vi "load_parameters.vi"(4 "Create Data Folder (T)":bool=TRUE, 5 "Set Up Projector and Camera (T)":bool=TRUE, 6 "additional loaded parameters to write":string[][](array[string]), 8 "error in (no error)":errorcluster, 9 "StimulusObject Parameters":variant, 10 "StimulusObjectClassInput":refnum<class "StimulusObject.lvclass">, 11 "Tags":string) -> (0 "error out":errorcluster, 2 "Computer Found":bool, 3 "Parameters":T1 {"FW_WormLengthSD" format="%#.6f"})   [LabVIEW 2019]
uses:
  Parameters.ctl
  StimulusObject.lvclass
  <vilib>/AdvancedString/Delimited String to 1D String Array.vi
  ParametersGlobal.vi
  <vilib>/Utility/file.llb/Write Delimited Spreadsheet (string).vi
  <vilib>/vision/driver/NI_Vision_Acquisition_Software.lvlib
  <vilib>/vision/NI_Vision_Development_Module.lvlib
panel:
  out "Cores Utilized":u32
  out "Camera Frame Rate":dbl
  # "Faux Worm Drawing"
  # "Tracking"
  # "Temporal Calibration"
  # "Stimulus Generation"
  # "Median Filtering"
  # "Experimental Settings"
  # "Camera and Projector Settings"
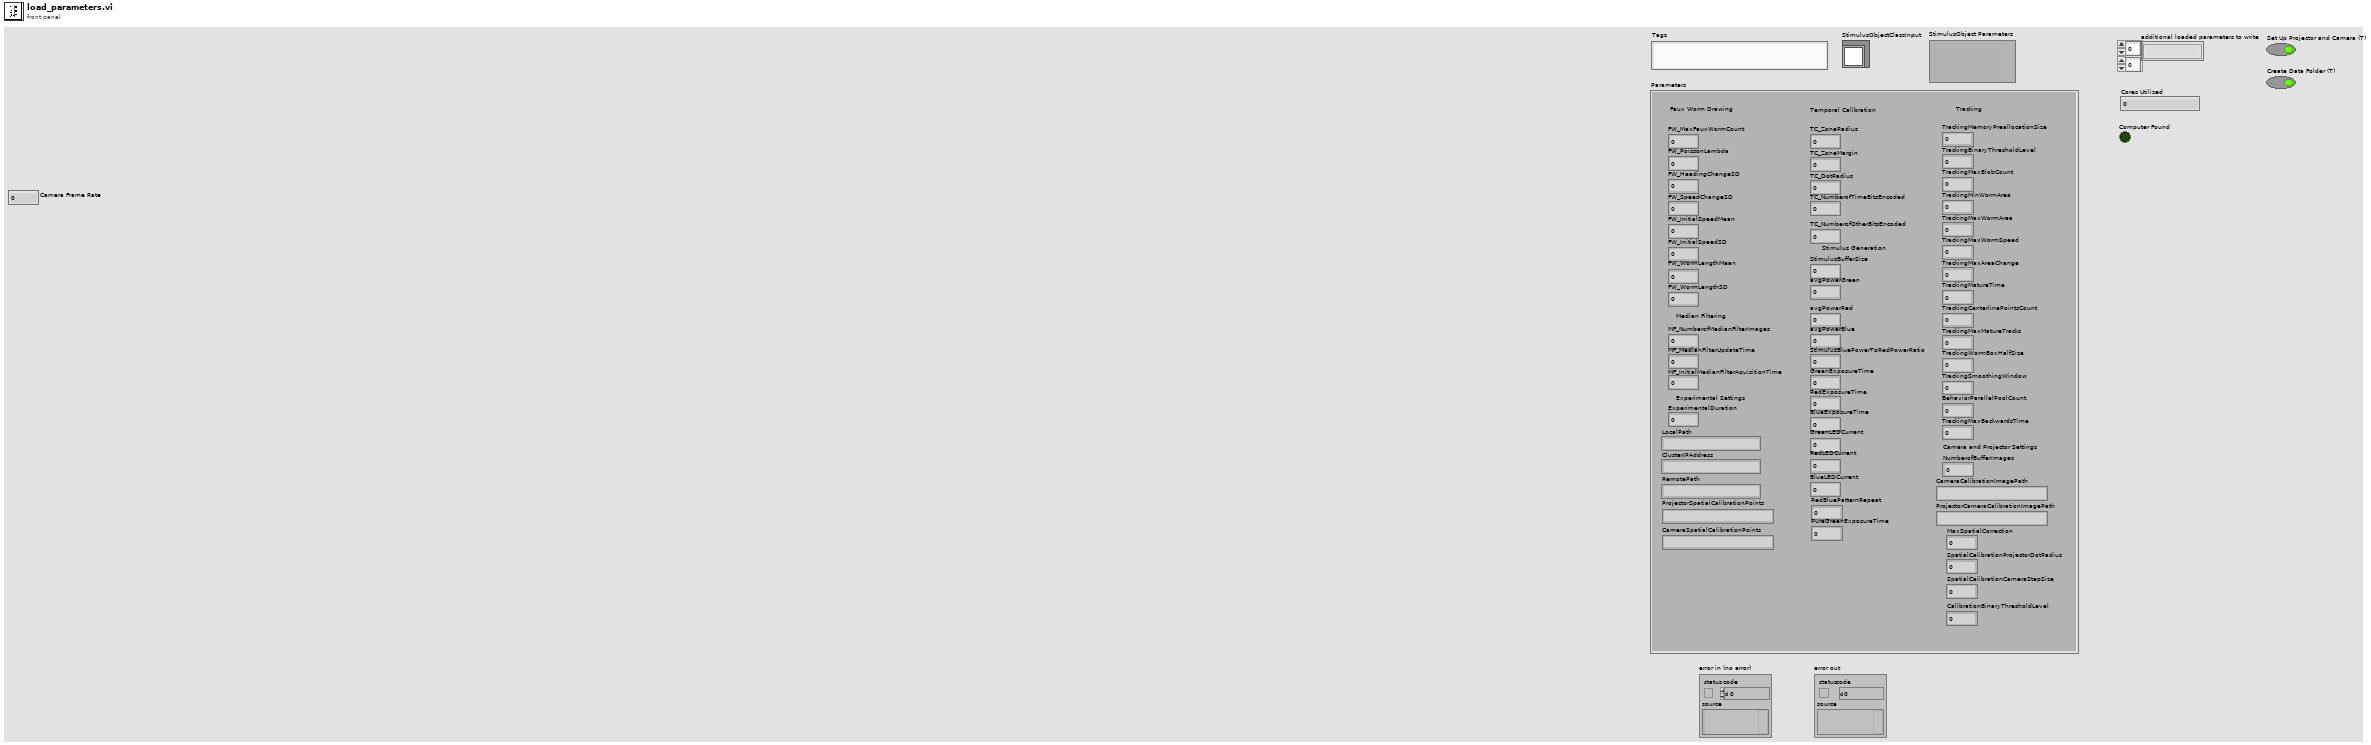
[diagram p1: front panel]
types:
  T1 = typedef "Parameters.ctl" = cluster{"FW_MaxFauxWormCount":i32, "FW_PoissonLambda":dbl, "FW_HeadingChangeSD":dbl, "FW_SpeedChangeSD":dbl, "FW_InitialSpeedMean":dbl, "FW_InitialSpeedSD":dbl, "FW_WormLengthMean":dbl, "FW_WormLengthSD":dbl, "MF_NumberofMedianFilterImages":i32, "MF_MedianFilterUpdateTime":i32, "MF_InitialMedianFilterAquisitionTime":dbl, "ExperimentalDuration":i32, "TC_ZoneRadius":i32, "TC_ZoneMargin":i32, "TC_DotRadius":dbl, "TC_NumberofTimeBitsEncoded":i32, "TC_NumberofOtherBitsEncoded":i32, "NumberofBufferImages":sgl, "CameraCalibrationImagePath":string, "ProjectorCameraCalibrationImagePath":string, "StimulusBufferSize":i32, "TrackingMemoryPreallocationSize":i32, "TrackingBinaryThresholdLevel":sgl, "TrackingMaxBlobCount":i32, "TrackingMinWormArea":dbl, "TrackingMaxWormArea":dbl, "TrackingMaxWormSpeed":dbl, "TrackingMaxAreaChange":dbl, "TrackingMatureTime":i32, "TrackingCenterlinePointsCount":i32, "TrackingMaxMatureTracks":i32, "TrackingWormBoxHalfSize":i32, "TrackingSmoothingWindow":i32, "BehaviorParallelPoolCount":i32, "LocalPath":string, "GreenExposureTime":i32, "RedExposureTime":i32, "BlueExposureTime":i32, "ClusterIPAddress":string, "RemotePath":string, "GreenLEDCurrent":u8, "RedLEDCurrent":u8, "BlueLEDCurrent":u8, "avgPowerGreen":sgl, "avgPowerRed":sgl, "avgPowerBlue":sgl, "StimulusBluePowerToRedPowerRatio":sgl, "TrackingMaxBackwardsTime":i32, "MaxSpatialCorrection":dbl, "ProjectorSpatialCalibrationPoints":string, "SpatialCalibrationProjectorDotRadius":i32, "SpatialCalibrationCameraStepSize":dbl, "CameraSpatialCalibrationPoints":string, "CalibrationBinaryThresholdLevel":dbl, "RedBluePatternRepeat":i32, "PureGreenExposureTime":i32}
  T2 = enum16{"open", "replace", "create", "open or create", "replace or create", "replace or create with confirmation"}
  T3 = typedef "IMAQ Image.ctl" = refnum<image>
  T4 = cluster{"Type":u32, "Version":u32, "Flags":u32, "SerialNumberHigh":u32, "SerialNumberLow":u32, "BusType":u32, "InterfaceName":string, "VendorName":string, "ModelName":string, "CameraFileName":string, "CameraAttributeURL":string}[]
  T5 = cluster{"Type":u32, "Version":u32, "Flags":u32, "SerialNumberHigh":u32, "SerialNumberLow":u32, "BusType":u32, "InterfaceName":string, "VendorName":string, "ModelName":string, "CameraFileName":string, "CameraAttributeURL":string}
  T6 = typedef "Image Type" = u32
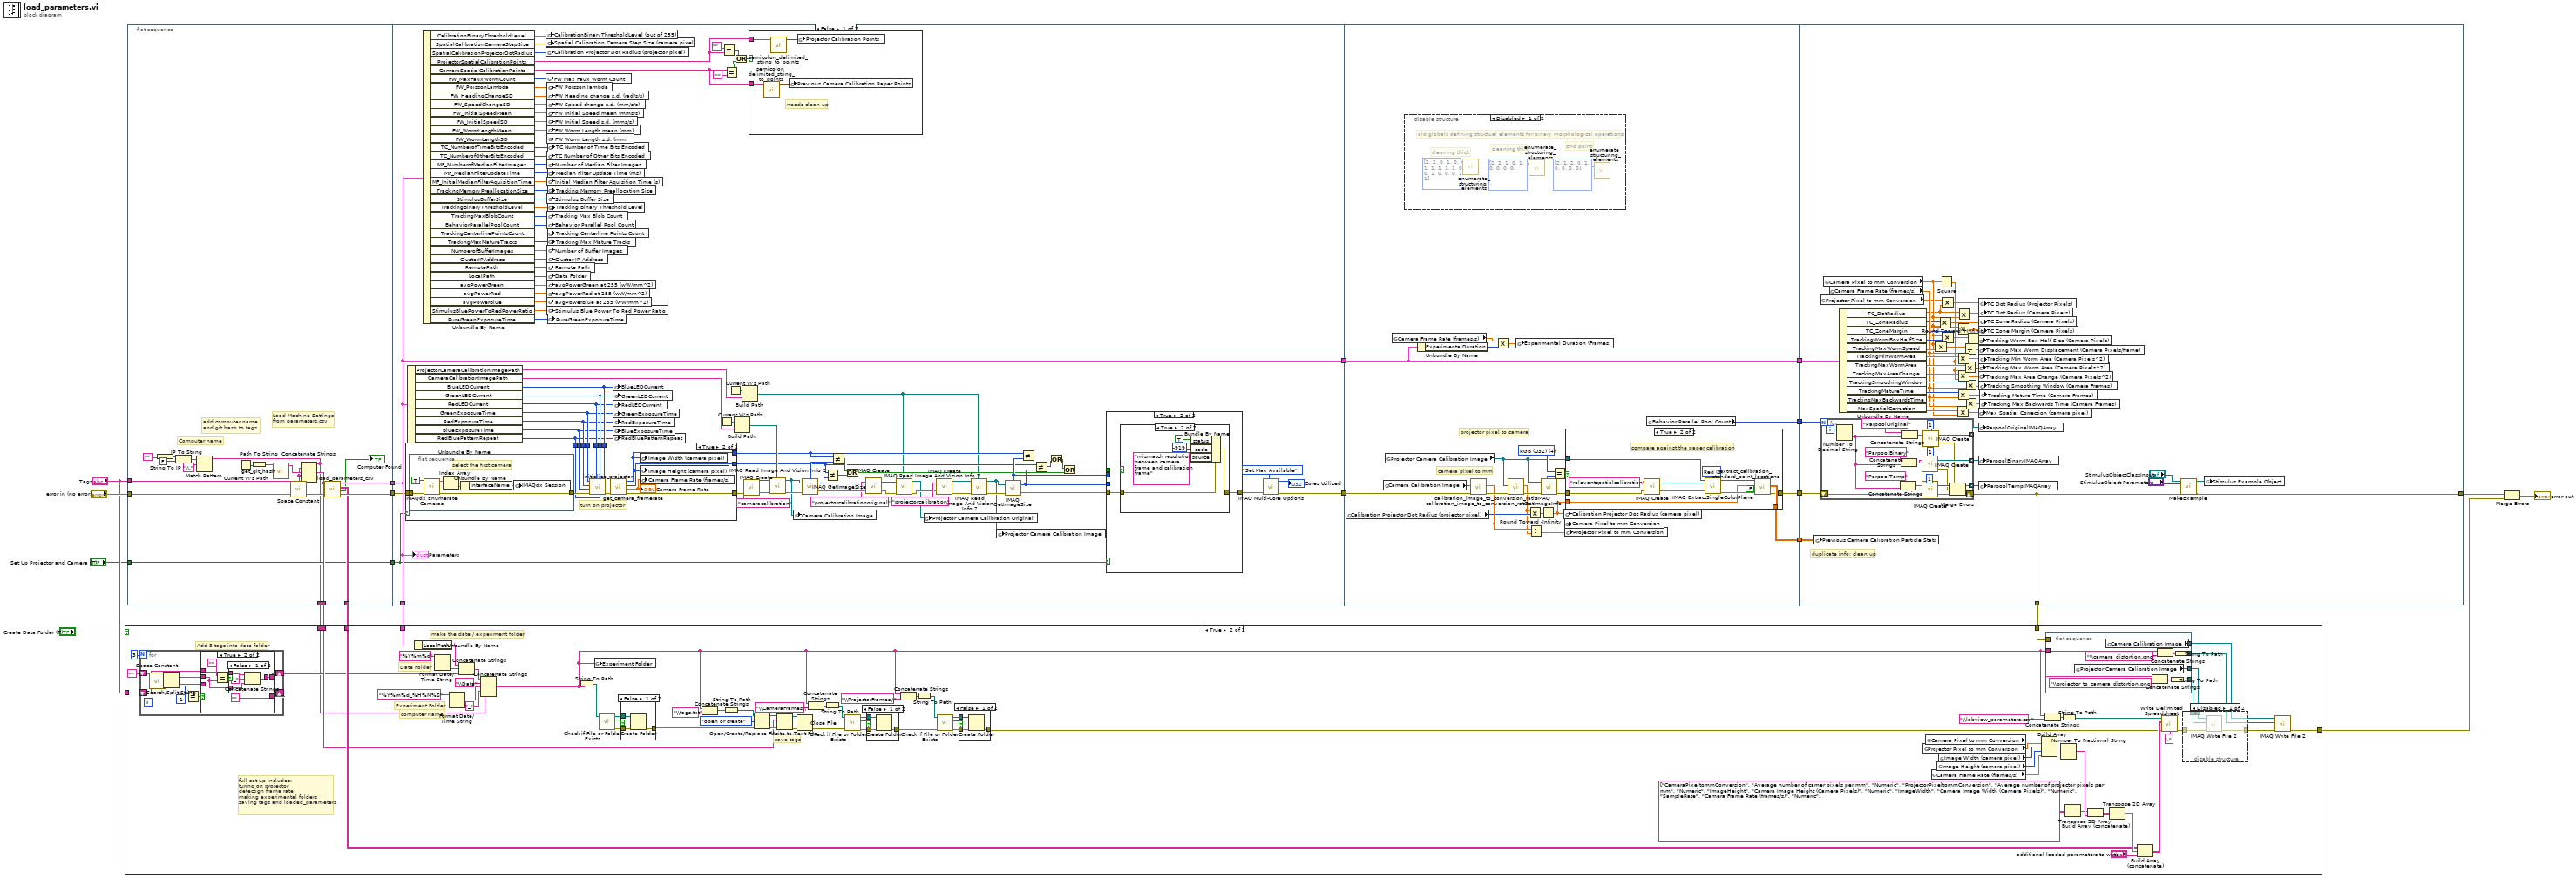
[diagram p0: block diagram]
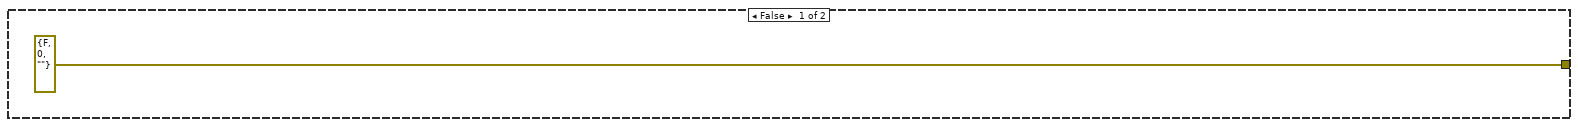
[diagram p2: hidden frame]
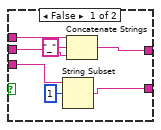
[diagram p7: hidden frame]
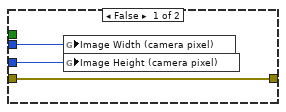
[diagram p10: hidden frame]
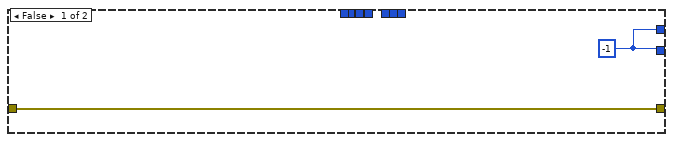
[diagram p12: hidden frame]
diagram:
  n1 = case shown="True" "Create Data Folder (T)" {
    tunnel: "Tags" -> [_ w92]
    tunnel: w12 -> [_ w41]
    tunnel: w11 -> [_ w39]
    tunnel: [errorcluster {"status"=FALSE, "code"=0, "source"=""} ("error out") w32] -> w8
    tunnel: w7 -> [_ w36]
    tunnel: w3 -> [_ w25]
    tunnel: w1 -> [_ w23]
    frame False {
    }
    frame True {
      # "computer name"
      # "full set up includes:\nturing on projector\ndetectign frame rate\nmaking experimental folders\nsaving tags and loaded_parameters"
      # "save tags"
      # "make the date / experiment folder"
      # "Experiment Folder"
      # "Date Folder"
      # "Add 3 tags into date folder"
      n2 = for {
        N: 3 -> [_]
        shift-right: [w119] -> _
        shift-left: w92 -> [w128]
        shift-right: [w121] -> w35
        shift-left: "" -> [w126]
        n3 = call <vilib>:"Space Constant.vi"() -> ("String"=w127:string)
        n4 = Search/Split String(string=w128, search string/char (-)=w127) -> (substring before match=w125:string, match + rest of string=w124:string, offset of match=w123:i32)  [unwired: 1 in]
        n5 = Equal?(x=w123, y=-1) -> (x = y?=w120:bool)
        n6 = case shown="True" w120 {
          tunnel: w126 -> [w129 w139]
          tunnel: w125 -> [w130 w136]
          tunnel: w124 -> [w131 _]
          tunnel: [w133 ""] -> w119
          tunnel: [w132 w138] -> w121
          frame False {
            n7 = String Subset(string=w131, offset (0)=1) -> (substring=w133:string)  [unwired: 1 in]
            n8 = Concatenate Strings(w129, "_", w130) -> (w132:string)
          }
          frame True {
            n9 = Equal?(x="", y=w136) -> (x = y?=w140:bool)
            n10 = case shown="False" w140 {
              tunnel: w139 -> [w143 w146]
              tunnel: [w144 w146] -> w138
              tunnel: w136 -> [w142 _]
              frame False {
                n11 = Concatenate Strings(w143, "_", w142) -> (w144:string)
              }
              frame True {
              }
            }
          }
        }
      }
      n12 = Unbundle By Name(w36) -> ("LocalPath"=w26:string)
      n13 = Format Date/Time String(time format string (%c)="%Y%m%d") -> (date/time string=w87:string)  [unwired: 2 in]
      n14 = Format Date/Time String(time format string (%c)="%Y%m%d_%H%M%S") -> (date/time string=w86:string)  [unwired: 2 in]
      n15 = Concatenate Strings(w26, w87, w35) -> (w88:string)
      n16 = Concatenate Strings(w88, "\\Data", w86, "_", w23) -> (w27:string)
      n17 = String To Path(string=w27) -> (path=w85:path)
      n18 = global write "ParametersGlobal.vi" "Experiment Folder"(w27) -> ()
      n19 = call <vilib>:"Check if File or Folder Exists.vi"("path"=w85) -> ("error out"=w89:errorcluster, "file or folder exists?"=w83:bool, "dup path"=w84:path)  [unwired: 8 in]
      n20 = case shown="False" w83 {
        tunnel: w84 -> [w117 _]
        tunnel: [w116 w118] -> w65
        tunnel: w89 -> [w115 w118]
        frame False {
          n21 = Create Folder(path (use dialog)=w117, error in=w115) -> (error out=w116:errorcluster)  [unwired: 1 in, 2 out]
        }
        frame True {
        }
      }
      n22 = Concatenate Strings(w27, "\\tags.txt" ("string")) -> (w69:string)
      n23 = String To Path(string=w69) -> (path=w72:path)
      n24 = Open/Create/Replace File(file path (use dialog)=w72, error in=w65, operation (0:open)=T2."open or create") -> (refnum out=w71:refnum<file>, error out=w70:errorcluster)  [unwired: 3 in, 1 out]
      n25 = Write to Text File(file (use dialog)=w71, text=w39, error in=w70) -> (refnum out=w73:refnum<file>, error out=w74:errorcluster)  [unwired: 1 in, 1 out]
      n26 = Close File(refnum=w73, error in=w74) -> (error out=w77:errorcluster)  [unwired: 1 out]
      n27 = Concatenate Strings(w27, "\\CameraFrames\\" ("string")) -> (w78:string)
      n28 = String To Path(string=w78) -> (path=w79:path)
      n29 = call <vilib>:"Check if File or Folder Exists.vi"("error in (no error)"=w77, "path"=w79) -> ("error out"=w80:errorcluster, "file or folder exists?"=w76:bool, "dup path"=w75:path)  [unwired: 7 in]
      n30 = case shown="False" w76 {
        tunnel: w75 -> [w113 _]
        tunnel: [w112 w114] -> w40
        tunnel: w80 -> [w111 w114]
        frame False {
          n31 = Create Folder(path (use dialog)=w113, error in=w111) -> (error out=w112:errorcluster)  [unwired: 1 in, 2 out]
        }
        frame True {
        }
      }
      n32 = Concatenate Strings(w27, "\\ProjectorFrames\\" ("string")) -> (w61:string)
      n33 = String To Path(string=w61) -> (path=w62:path)
      n34 = call <vilib>:"Check if File or Folder Exists.vi"("error in (no error)"=w40, "path"=w62) -> ("error out"=w63:errorcluster, "file or folder exists?"=w60:bool, "dup path"=w59:path)  [unwired: 7 in]
      n35 = case shown="False" w60 {
        tunnel: w59 -> [w109 _]
        tunnel: [w108 w110] -> w38
        tunnel: w63 -> [w107 w110]
        frame False {
          n36 = Create Folder(path (use dialog)=w109, error in=w107) -> (error out=w108:errorcluster)  [unwired: 1 in, 2 out]
        }
        frame True {
        }
      }
      n37 = global read "ParametersGlobal.vi" "Projector Pixel to mm Conversion"() -> (w49:sgl)
      n38 = global read "ParametersGlobal.vi" "Camera Pixel to mm Conversion"() -> (w48:sgl)
      n39 = global read "ParametersGlobal.vi" "Camera Frame Rate (frames/s)"() -> (w64:sgl)
      n40 = global read "ParametersGlobal.vi" "Image Height (camera pixel)"() -> (w51:i32)
      n41 = global read "ParametersGlobal.vi" "Image Width (camera pixel)"() -> (w50:i32)
      n42 = Build Array(w48, w49, w50, w51, w64) -> (w52:sgl[])
      n43 = Concatenate Strings(w27, "\\labview_parameters.csv" ("string")) -> (w46:string)
      n44 = flat-sequence {
        tunnel: [w106] -> w31
        tunnel: [w105] -> w30
        tunnel: [w100] -> w29
        tunnel: [w99] -> w28
        tunnel: w27 -> [w98]
        tunnel: w25 -> [_]
        frame #0 {
          n45 = global read "ParametersGlobal.vi" "Projector Camera Calibration Image"() -> (w106:T3)
          n46 = global read "ParametersGlobal.vi" "Camera Calibration Image"() -> (w105:T3)
          n47 = Concatenate Strings(w98, "\\projector_to_camera_distortion.png" ("string")) -> (w102:string)
          n48 = Concatenate Strings(w98, "\\camera_distortion.png" ("string")) -> (w104:string)
          n49 = String To Path(string=w102) -> (path=w100:path)
          n50 = String To Path(string=w104) -> (path=w99:path)
        }
      }
      n51 = Number To Fractional String(number=w52) -> (F-format string=w54:string[])  [unwired: 3 in]
      n52 = String To Path(string=w46) -> (path=w47:path)
      n53 = Transpose 2D Array(2D array=string[][] [["CameraPixeltommConversion", "Average number of camer pixels per mm", "Numeric"], ["ProjectorPixeltommConversion", "Average number of projector pixels per mm", "Numeric"], ["ImageHeight", "Camera Image Height (Camera Pixels)", "Numeric"], ["ImageWidth", "Camera Image Width (Camera Pixels)", "Numeric"], ["SampleRate", "Camera Frame Rate (frames/s)", "Numeric"]]) -> (transposed array=w53:string[][])
      n54 = Build Array (concatenate)(w53, w54) -> (w55:string[][])
      n55 = Transpose 2D Array(2D array=w55) -> (transposed array=w56:string[][])
      n56 = Build Array (concatenate)(w41, w56, "additional loaded parameters to write") -> (w58:string[][])
      n57 = call-poly <vilib>:"Write Delimited Spreadsheet.vi"("file path (dialog if empty)"=w47, "2D data"=w58, "error in (no error)"=w38, "delimiter (\\t)"="," ("delimiter (\\t)")) -> ("error out"=w34:errorcluster)  [unwired: 10 in, 1 out]
      n58 = disable-structure shown="Disabled" {
        disable-tunnel: w34 -> [w96 w97]
        disable-tunnel: [w95 w97] -> w33
        disable-tunnel: w31 -> [w94 _]
        disable-tunnel: w29 -> [w93 _]
        frame Disabled {
          n59 = call-poly "IMAQ Write File 2"("error in (no error)"=w96, "File Path"=w93, "Image"=w94) -> ("error out"=w95:errorcluster)  [unwired: 7 in, 1 out]
        }
        frame Enabled {
        }
      }
      n60 = call-poly "IMAQ Write File 2"("error in (no error)"=w33, "File Path"=w28, "Image"=w30) -> ("error out"=w32:errorcluster)  [unwired: 7 in, 1 out]
    }
  }
  n61 = flat-sequence {
    tunnel: [w164] -> w20
    tunnel: "error in (no error)" -> [w150]
    tunnel: [w151] -> w19
    tunnel: "Tags" -> [w156]
    tunnel: [w153] -> w12
    tunnel: [w152] -> w11
    tunnel: [w149] -> w6
    tunnel: "Set Up Projector and Camera (T)" -> [w149]
    tunnel: [w147] -> w1
    tunnel: w20 -> [w222]
    tunnel: [w213] -> w18
    tunnel: w19 -> [w223]
    tunnel: [w223] -> w15
    tunnel: [w223] -> w7
    tunnel: w6 -> [w199]
    tunnel: w18 -> [w313]
    tunnel: [w301] -> w17
    tunnel: [w309] -> w16
    tunnel: w15 -> [w309]
    tunnel: [w310] -> w14
    tunnel: [w298] -> w2
    tunnel: w17 -> [w352]
    tunnel: w16 -> [w373]
    tunnel: w14 -> [w351]
    tunnel: [w340] -> w10
    tunnel: [w344] -> w3
    tunnel: w2 -> [w343]
    frame #0 {
      # "add computer name \nand git hash to tags"
      # "Computer name"
      # "Load Machine Settings\nfrom parameters.csv"
      n62 = String To IP(1:"") -> (0:w163:u32)
      n63 = IP To String(1:FALSE, 2:w163) -> (0:w160:string)
      n64 = Match Pattern(string=w160, regular expression="\\.") -> (before substring=w147:string)  [unwired: 1 in, 3 out]
      n65 = Current VI's Path() -> (path=w158:path)
      n66 = Path To String(path=w158) -> (string=w157:string)
      n67 = call "get_git_hash.vi"("VI folder"=w157) -> ("github hash"=w155:string)  [unwired: 10 in]
      n68 = call <vilib>:"Space Constant.vi"() -> ("String"=w154:string)
      n69 = Concatenate Strings(w147, w154, w155, w154, w156) -> (w152:string)
      n70 = call "load_parameters_csv.vi"("error in (no error)"=w150, "Tags In"=w152) -> ("error out"=w164:errorcluster, "Computer Found"=→"Computer Found":bool, "Loaded Params"=w153:string[][], "Parameters Out"=w151:T1)  [unwired: 6 in]
    }
    frame #1 {
      n71 = Unbundle By Name(w223) -> ("ProjectorCameraCalibrationImagePath"=w193:string, "CameraCalibrationImagePath"=w245:string, "BlueLEDCurrent"=w172:u8, "GreenLEDCurrent"=w171:u8, "RedLEDCurrent"=w170:u8, "GreenExposureTime"=w169:i32, "RedExposureTime"=w168:i32, "BlueExposureTime"=w167:i32, "RedBluePatternRepeat"=w166:i32)
      n72 = case shown="True" w199 {
        tunnel: w222 -> [w272 w277]
        tunnel: [w272 w284] -> w221
        tunnel: w169 -> [_ w283]
        tunnel: w168 -> [_ w282]
        tunnel: w167 -> [_ w281]
        tunnel: w170 -> [_ w280]
        tunnel: w172 -> [_ w279]
        tunnel: w171 -> [_ w278]
        tunnel: [w271 w275] -> w192
        tunnel: [w271 w274] -> w191
        tunnel: w166 -> [_ w273]
        frame False {
          w271 = -1 ("Image Width (camera pixel)")
        }
        frame True {
          # "turn on projector"
          n73 = flat-sequence {
            tunnel: w277 -> [w289]
            tunnel: [w288] -> w276
            frame #0 {
              # "select the first camera"
              n74 = call <vilib>:"IMAQdx Enumerate Cameras.vi"("error in"=w289, "Connected Only? (Yes)"=TRUE) -> ("error out"=w288:errorcluster, "Camera Information Array"=w292:T4)  [unwired: 8 in]
              n75 = Index Array(array=w292) -> (element=w291:T5)  [unwired: 1 in]
              n76 = Unbundle By Name(w291) -> ("InterfaceName"=w287:string)
              n77 = global write "ParametersGlobal.vi" "IMAQdx Session"(w287) -> ()
            }
          }
          n78 = call "initialize_projector.vi"("BlueCurrent"=w279, "RedBluePatternRepeat"=w273, "GreenCurrent"=w278, "RedCurrent"=w280, "error in"=w276, "blue exp_time_us"=w281, "red exp_time_us"=w282, "green exp_time_us"=w283) -> ("error out"=w285:errorcluster)  [unwired: 3 in]
          n79 = call "get_camera_framerate.vi"("error in"=w285) -> ("error out"=w284:errorcluster, "Camera Frame Rate"=w286:dbl, "Y Resolution"=w274:i32, "X Resolution"=w275:i32)  [unwired: 7 in]
          "Camera Frame Rate" <- w286
          n80 = global write "ParametersGlobal.vi" "Image Width (camera pixel)"(w275) -> ()
          n81 = global write "ParametersGlobal.vi" "Image Height (camera pixel)"(w274) -> ()
          n82 = global write "ParametersGlobal.vi" "Camera Frame Rate (frames/s)"(w286) -> ()
        }
      }
      n83 = Unbundle By Name(w223) -> ("CalibrationBinaryThresholdLevel"=w173:dbl, "SpatialCalibrationCameraStepSize"=w187:dbl, "SpatialCalibrationProjectorDotRadius"=w188:i32, "ProjectorSpatialCalibrationPoints"=w189:string, "CameraSpatialCalibrationPoints"=w174:string, "FW_MaxFauxWormCount"=w235:i32, "FW_PoissonLambda"=w236:dbl, "FW_HeadingChangeSD"=w237:dbl, "FW_SpeedChangeSD"=w238:dbl, "FW_InitialSpeedMean"=w239:dbl, "FW_InitialSpeedSD"=w240:dbl, "FW_WormLengthMean"=w241:dbl, "FW_WormLengthSD"=w242:dbl, "TC_NumberofTimeBitsEncoded"=w243:i32, "TC_NumberofOtherBitsEncoded"=w244:i32, "MF_NumberofMedianFilterImages"=w234:i32, "MF_MedianFilterUpdateTime"=w233:i32, "MF_InitialMedianFilterAquisitionTime"=w232:dbl, "TrackingMemoryPreallocationSize"=w231:i32, "StimulusBufferSize"=w230:i32, "TrackingBinaryThresholdLevel"=w229:sgl, "TrackingMaxBlobCount"=w228:i32, "BehaviorParallelPoolCount"=w227:i32, "TrackingCenterlinePointsCount"=w226:i32, "TrackingMaxMatureTracks"=w225:i32, "NumberofBufferImages"=w224:sgl, "ClusterIPAddress"=w220:string, "RemotePath"=w219:string, "LocalPath"=w218:string, "avgPowerGreen"=w214:sgl, "avgPowerRed"=w215:sgl, "avgPowerBlue"=w216:sgl, "StimulusBluePowerToRedPowerRatio"=w217:sgl, "PureGreenExposureTime"=w165:i32)
      n84 = global write "ParametersGlobal.vi" "CalibrationBinaryThresholdLevel (out of 255)"(w173) -> ()
      n85 = global write "ParametersGlobal.vi" "Spatial Calibration Camera Step Size (camera pixel)"(w187) -> ()
      n86 = global write "ParametersGlobal.vi" "Calibration Projector Dot Radius (projector pixel)"(w188) -> ()
      n87 = global write "ParametersGlobal.vi" "FW Max Faux Worm Count"(w235) -> ()
      n88 = global write "ParametersGlobal.vi" "FW Poisson lambda"(w236) -> ()
      n89 = global write "ParametersGlobal.vi" "FW Heading change s.d. (rad/s/s)"(w237) -> ()
      n90 = global write "ParametersGlobal.vi" "FW Speed change s.d. (mm/s/s)"(w238) -> ()
      n91 = global write "ParametersGlobal.vi" "FW Initial Speed mean (mms/s)"(w239) -> ()
      n92 = global write "ParametersGlobal.vi" "FW Initial Speed s.d. (mms/s)"(w240) -> ()
      n93 = global write "ParametersGlobal.vi" "FW Worm Length mean (mm)"(w241) -> ()
      n94 = global write "ParametersGlobal.vi" "FW Worm Length s.d. (mm)"(w242) -> ()
      n95 = global write "ParametersGlobal.vi" "TC Number of Other Bits Encoded"(w244) -> ()
      n96 = global write "ParametersGlobal.vi" "Number of Median Filter Images"(w234) -> ()
      n97 = global write "ParametersGlobal.vi" "Initial Median Filter Aquisition Time (s)"(w232) -> ()
      n98 = global write "ParametersGlobal.vi" "Stimulus Buffer Size"(w230) -> ()
      n99 = global write "ParametersGlobal.vi" "Tracking Max Blob Count"(w228) -> ()
      n100 = global write "ParametersGlobal.vi" "Behavior Parallel Pool Count"(w227) -> ()
      n101 = global write "ParametersGlobal.vi" "Number of Buffer Images"(w224) -> ()
      n102 = global write "ParametersGlobal.vi" "Cluster IP Address"(w220) -> ()
      n103 = global write "ParametersGlobal.vi" "Remote Path"(w219) -> ()
      n104 = global write "ParametersGlobal.vi" "Data Folder"(w218) -> ()
      n105 = global write "ParametersGlobal.vi" "avgPowerGreen at 255 (wW/mm^2)"(w214) -> ()
      n106 = global write "ParametersGlobal.vi" "avgPowerRed at 255 (wW/mm^2)"(w215) -> ()
      n107 = global write "ParametersGlobal.vi" "avgPowerBlue at 255 (wW/mm^2)"(w216) -> ()
      n108 = global write "ParametersGlobal.vi" "Stimulus Blue Power To Red Power Ratio"(w217) -> ()
      n109 = global write "ParametersGlobal.vi" "TC Number of Time Bits Encoded"(w243) -> ()
      n110 = global write "ParametersGlobal.vi" "Median Filter Update Time (ms)"(w233) -> ()
      n111 = global write "ParametersGlobal.vi" "Tracking Memory Preallocation Size"(w231) -> ()
      n112 = global write "ParametersGlobal.vi" "Tracking Binary Threshold Level"(w229) -> ()
      n113 = global write "ParametersGlobal.vi" "Tracking Centerline Points Count"(w226) -> ()
      n114 = global write "ParametersGlobal.vi" "Tracking Max Mature Tracks"(w225) -> ()
      n115 = global write "ParametersGlobal.vi" "PureGreenExposureTime"(w165) -> ()
      n116 = global write "ParametersGlobal.vi" "BlueLEDCurrent"(w172) -> ()
      n117 = global write "ParametersGlobal.vi" "GreenLEDCurrent"(w171) -> ()
      n118 = global write "ParametersGlobal.vi" "RedLEDCurrent"(w170) -> ()
      n119 = global write "ParametersGlobal.vi" "GreenExposureTime"(w169) -> ()
      n120 = global write "ParametersGlobal.vi" "RedExposureTime"(w168) -> ()
      n121 = global write "ParametersGlobal.vi" "BlueExposureTime"(w167) -> ()
      n122 = global write "ParametersGlobal.vi" "RedBluePatternRepeat"(w166) -> ()
      n123 = Current VI's Path() -> (path=w250:path)
      n124 = Equal?(x="", y=w189) -> (x = y?=w177:bool)
      n125 = Equal?(x=w174, y="") -> (x = y?=w176:bool)
      n126 = Current VI's Path() -> (path=w254:path)
      n127 = Or(x=w177, y=w176) -> (x .or. y?=w175:bool)
      n128 = Build Path(base path=w250, name or relative path=w245) -> (appended path=w247:path)
      n129 = Build Path(base path=w254, name or relative path=w193) -> (appended path=w180:path)
      n130 = call "IMAQ Create"("Image Name"="cameracalibration", "error in (no error)"=w221) -> ("New Image"=w249:T3, "error out"=w248:errorcluster)  [unwired: 3 in]
      n131 = case shown="False" w175 {
        tunnel: w189 -> [w258 _]
        tunnel: w174 -> [w256 _]
        frame False {
          # "needs clean up"
          n132 = call "semicolon_delimited_string_to_points.vi"("delimited string"=w256) -> ("Array"=w255:cluster{"X":dbl, "Y":dbl}[])  [unwired: 10 in]
          n133 = call "semicolon_delimited_string_to_points.vi"("delimited string"=w258) -> ("Array"=w257:cluster{"X":dbl, "Y":dbl}[])  [unwired: 10 in]
          n134 = global write "ParametersGlobal.vi" "Previous Camera Calibration Paper Points"(w255) -> ()
          n135 = global write "ParametersGlobal.vi" "Projector Calibration Points"(w257) -> ()
        }
        frame True {
        }
      }
      n136 = call "IMAQ Read Image And Vision Info 2"("File Path"=w247, "error in (no error)"=w248, "Image"=w249) -> ("error out"=w210:errorcluster, "Image Out"=w207:T3)  [unwired: 6 in, 1 out]
      n137 = global write "ParametersGlobal.vi" "Camera Calibration Image"(w207) -> ()
      n138 = call "IMAQ GetImageSize"("Image"=w207, "error in (no error)"=w210) -> ("Y Resolution"=w208:i32, "X Resolution"=w209:i32, "error out"=w185:errorcluster)  [unwired: 2 in]
      n139 = Not Equal?(x=w191, y=w208) -> (x != y?=w204:bool)
      n140 = Not Equal?(x=w192, y=w209) -> (x != y?=w203:bool)
      n141 = Or(x=w203, y=w204) -> (x .or. y?=w186:bool)
      n142 = call "IMAQ Create"("Image Name"="projectorcalibrationoriginal", "error in (no error)"=w185) -> ("New Image"=w182:T3, "error out"=w183:errorcluster)  [unwired: 3 in]
      n143 = call "IMAQ Read Image And Vision Info 2"("File Path"=w180, "error in (no error)"=w183, "Image"=w182) -> ("error out"=w181:errorcluster, "Image Out"=w179:T3)  [unwired: 6 in, 1 out]
      n144 = global write "ParametersGlobal.vi" "Projector Camera Calibration Original"(w179) -> ()
      n145 = call "IMAQ Create"("Image Name"="projectorcalibration", "error in (no error)"=w181) -> ("New Image"=w252:T3, "error out"=w251:errorcluster)  [unwired: 3 in]
      n146 = call "IMAQ Read Image And Vision Info 2"("File Path"=w180, "error in (no error)"=w251, "Image"=w252) -> ("error out"=w206:errorcluster, "Image Out"=w205:T3)  [unwired: 6 in, 1 out]
      n147 = global write "ParametersGlobal.vi" "Projector Camera Calibration Image"(w205) -> ()
      n148 = call "IMAQ GetImageSize"("Image"=w205, "error in (no error)"=w206) -> ("Y Resolution"=w196:i32, "X Resolution"=w195:i32, "error out"=w198:errorcluster)  [unwired: 2 in]
      n149 = Not Equal?(x=w192, y=w195) -> (x != y?=w202:bool)
      n150 = Not Equal?(x=w191, y=w196) -> (x != y?=w201:bool)
      n151 = Or(x=w202, y=w201) -> (x .or. y?=w200:bool)
      n152 = Or(x=w200, y=w186) -> (x .or. y?=w194:bool)
      n153 = case shown="True" w199 {
        tunnel: w198 -> [w261 w263]
        tunnel: [w261 w262] -> w197
        tunnel: w196 -> [w260 _]
        tunnel: w195 -> [w259 _]
        tunnel: w194 -> [_ w264]
        frame False {
          n154 = global write "ParametersGlobal.vi" "Image Width (camera pixel)"(w259) -> ()
          n155 = global write "ParametersGlobal.vi" "Image Height (camera pixel)"(w260) -> ()
        }
        frame True {
          n156 = case shown="True" w264 {
            tunnel: w263 -> [w265 w267]
            tunnel: [w265 w266] -> w262
            frame False {
              # "all resolutions match"
            }
            frame True {
              n157 = Bundle By Name(cluster=w267, "status"=TRUE, "code"=-919, "source"="mismatch resolution between camera frame and calibration frame") -> (w266:errorcluster)
            }
          }
        }
      }
      n158 = call "IMAQ Multi-Core Options"("Get/Set Number of Cores (Get)"=enum32{"Get", "Set", "Set Max Available"}."Set Max Available", "error in (no error)"=w197) -> ("error out"=w213:errorcluster, "Cores Utilized"=→"Cores Utilized":u32)  [unwired: 8 in]
      "Parameters" <- w223
    }
    frame #2 {
      w302 = T6 4 items=["Grayscale (U8)", "Grayscale (I16)", "Grayscale (SGL)", "Complex (CSG)", "RGB (U32)", "HSL (U32)", "RGB (U64)", "Grayscale (U16)"] ("Image Type")
      # "projector pixel to camera"
      # "camera pixel to mm"
      n159 = global read "ParametersGlobal.vi" "Calibration Projector Dot Radius (projector pixel)"() -> (w296:i32)
      n160 = global read "ParametersGlobal.vi" "Camera Calibration Image"() -> (w312:T3)
      n161 = global read "ParametersGlobal.vi" "Projector Camera Calibration Image"() -> (w297:T3)
      n162 = global read "ParametersGlobal.vi" "Camera Frame Rate (frames/s)"() -> (w308:sgl)
      n163 = disable-structure shown="Disabled" {
        frame Disabled {
          # "old globals defining structual elements for binary morphological operations"
          # "End point"
          # "cleaning thin"
          # "cleaning thick"
          n164 = call "enumerate_structuring_elements.vi"("Structuring Elements"=i32[][][] [[[2, 2, 0], [1, 0, 1], [1, 1, 1]], [[1, 0, 0], [1, 0, 0], [0, 1, 1]]]) -> ()  [unwired: 4 in, 1 out]
          n165 = call "enumerate_structuring_elements.vi"("Structuring Elements"=i32[][][] [[[2, 2, 1], [0, 1, 0], [0, 0, 0]]]) -> ()  [unwired: 4 in, 1 out]
          n166 = call "enumerate_structuring_elements.vi"("Structuring Elements"=i32[][][] [[[2, 1, 2], [0, 1, 0], [0, 0, 0]]]) -> ()  [unwired: 4 in, 1 out]
        }
        frame Enabled {
        }
      }
      n167 = Unbundle By Name(w309) -> ("ExperimentalDuration"=w307:i32)
      n168 = call "calibration_image_to_conversion_ratio.vi"("error in (no error)"=w313, "Calibration Image"=w312) -> ("error out"=w314:errorcluster, "conversion ratio"=w305:dbl)  [unwired: 8 in]
      n169 = Multiply(x=w308, y=w307) -> (x*y=w306:sgl)
      n170 = call "calibration_image_to_conversion_ratio.vi"("error in (no error)"=w314, "Calibration Image"=w297) -> ("error out"=w304:errorcluster, "conversion ratio"=w295:dbl)  [unwired: 8 in]
      n171 = global write "ParametersGlobal.vi" "Experimental Duration (Frames)"(w306) -> ()
      n172 = Multiply(x=w295, y=w296) -> (x*y=w294:dbl)
      n173 = Divide(x=w305, y=w295) -> (x/y=w311:dbl)
      n174 = Round Toward -Infinity(1:w294) -> (0:w293:dbl)
      n175 = call "IMAQ GetImageInfo"("error in (no error)"=w304, "Image"=w297) -> ("error out"=w300:errorcluster, "Image Type"=w303:T6)  [unwired: 2 in, 6 out]
      n176 = Equal?(x=w302, y=w303) -> (x = y?=w299:bool)
      n177 = global write "ParametersGlobal.vi" "Calibration Projector Dot Radius (camera pixel)"(w293) -> ()
      n178 = global write "ParametersGlobal.vi" "Camera Pixel to mm Conversion"(w305) -> ()
      n179 = global write "ParametersGlobal.vi" "Projector Pixel to mm Conversion"(w311) -> ()
      n180 = case shown="True" w299 {
        tunnel: [w315 w321] -> w301
        tunnel: w300 -> [w315 w325]
        tunnel: w297 -> [_ w322]
        tunnel: [_ w323] -> w298
        tunnel: w293 -> [_ w320]
        frame False {
        }
        frame True {
          w317 = 0 items=["Red", "Green", "Blue", "Hue", "Saturation", "Luminance", "Value", "Intensity"] ("Color Plane")
          # "compare against the paper calibration"
          n181 = call "IMAQ Create"("Image Name"="relevantspatialcalibration", "error in (no error)"=w325) -> ("New Image"=w318:T3, "error out"=w319:errorcluster)  [unwired: 3 in]
          n182 = call "IMAQ ExtractSingleColorPlane"("Color Plane"=w317, "error in (no error)"=w319, "Image Dst"=w318, "Image Src"=w322) -> ("error out"=w326:errorcluster, "Image Dst Out"=w327:T3)  [unwired: 6 in]
          n183 = call "extract_calibration_standard_point_locations.vi"("error in (no error)"=w326, "Agar (T) Paper (F)"=FALSE, "expected dot radius (camera pixels)"=w320, "Image Src"=w327) -> ("error out"=w321:errorcluster, "Particle Measurements (Pixels)"=w323:dbl[][])  [unwired: 5 in, 1 out]
        }
      }
      n184 = global read "ParametersGlobal.vi" "Behavior Parallel Pool Count"() -> (w310:i32)
    }
    frame #3 {
      # "duplicate info: clean up"
      n185 = global write "ParametersGlobal.vi" "Previous Camera Calibration Particle Stats"(w343) -> ()
      n186 = global read "ParametersGlobal.vi" "Projector Pixel to mm Conversion"() -> (w332:sgl)
      n187 = for {
        N: w351 -> [_]
        shift-right: [w386] -> w344
        shift-left: w352 -> [w377]
        tunnel: [w390] -> w353 mode=indexing
        tunnel: [w385] -> w354 mode=indexing
        tunnel: [w382] -> w355 mode=indexing
        i -> [w387]
        n188 = Number To Decimal String(number=w387) -> (decimal integer string=w381:string)  [unwired: 1 in]
        n189 = Concatenate Strings("ParpoolTemp", w381) -> (w384:string)
        n190 = Concatenate Strings("ParpoolBinary", w381) -> (w388:string)
        n191 = Concatenate Strings("ParpoolOriginal", w381) -> (w391:string)
        n192 = call "IMAQ Create"("Border Size"=1, "Image Name"=w388) -> ("New Image"=w385:T3, "error out"=w379:errorcluster)  [unwired: 3 in]
        n193 = call "IMAQ Create"("Border Size"=1, "Image Name"=w384, "error in (no error)"=w377) -> ("New Image"=w382:T3, "error out"=w380:errorcluster)  [unwired: 2 in]
        n194 = call "IMAQ Create"("Border Size"=1, "Image Name"=w391) -> ("New Image"=w390:T3, "error out"=w378:errorcluster)  [unwired: 3 in]
        n195 = Merge Errors(w378, w379, w380) -> (w386:errorcluster)
      }
      n196 = global read "ParametersGlobal.vi" "Camera Pixel to mm Conversion"() -> (w337:sgl)
      n197 = global read "ParametersGlobal.vi" "Camera Frame Rate (frames/s)"() -> (w347:sgl)
      n198 = Unbundle By Name(w373) -> ("TC_DotRadius"=w333:dbl, "TC_ZoneRadius"=w339:i32, "TC_ZoneMargin"=w338:i32, "TrackingWormBoxHalfSize"=w362:i32, "TrackingMaxWormSpeed"=w365:dbl, "TrackingMinWormArea"=w372:dbl, "TrackingMaxWormArea"=w371:dbl, "TrackingMaxAreaChange"=w368:dbl, "TrackingSmoothingWindow"=w359:i32, "TrackingMatureTime"=w357:i32, "TrackingMaxBackwardsTime"=w348:i32, "MaxSpatialCorrection"=w342:dbl)
      n199 = Multiply(x=w337, y=w365) -> (x*y=w364:dbl)
      n200 = Multiply(x=w339, y=w337) -> (x*y=w335:sgl)
      n201 = Square(x=w337) -> (x^2=w367:sgl)
      n202 = Multiply(x=w332, y=w333) -> (x*y=w331:dbl)
      n203 = Multiply(x=w337, y=w362) -> (x*y=w361:sgl)
      n204 = Multiply(x=w342, y=w337) -> (x*y=w341:dbl)
      n205 = Multiply(x=w337, y=w338) -> (x*y=w334:sgl)
      n206 = Multiply(x=w372, y=w367) -> (x*y=w370:dbl)
      n207 = Multiply(x=w368, y=w367) -> (x*y=w366:dbl)
      n208 = Multiply(x=w357, y=w347) -> (x*y=w356:sgl)
      n209 = Multiply(x=w333, y=w337) -> (x*y=w336:dbl)
      n210 = Multiply(x=w371, y=w367) -> (x*y=w369:dbl)
      n211 = Divide(x=w364, y=w347) -> (x/y=w363:dbl)
      n212 = Multiply(x=w359, y=w347) -> (x*y=w358:sgl)
      n213 = Multiply(x=w348, y=w347) -> (x*y=w346:sgl)
      n214 = Round Toward +Infinity(x=w361) -> (ceil(x): smallest int >= x=w360:sgl)
      n215 = global write "ParametersGlobal.vi" "Tracking Worm Box Half Size (Camera Pixels)"(w360) -> ()
      n216 = global write "ParametersGlobal.vi" "Tracking Max Worm Displacement (Camera Pixels/frame)"(w363) -> ()
      n217 = global write "ParametersGlobal.vi" "Tracking Max Worm Area (Camera Pixels^2)"(w369) -> ()
      n218 = global write "ParametersGlobal.vi" "Tracking Max Area Change (Camera Pixels^2)"(w366) -> ()
      n219 = global write "ParametersGlobal.vi" "Max Spatial Correction (camera pixel)"(w341) -> ()
      n220 = global write "ParametersGlobal.vi" "ParpoolOriginalIMAQArray"(w353) -> ()
      n221 = global write "ParametersGlobal.vi" "ParpoolBinaryIMAQArray"(w354) -> ()
      n222 = global write "ParametersGlobal.vi" "TC Dot Radius (Projector Pixels)"(w331) -> ()
      n223 = global write "ParametersGlobal.vi" "TC Dot Radius (Camera Pixels)"(w336) -> ()
      n224 = global write "ParametersGlobal.vi" "TC Zone Radius (Camera Pixels)"(w335) -> ()
      n225 = global write "ParametersGlobal.vi" "TC Zone Margin (Camera Pixels)"(w334) -> ()
      n226 = global write "ParametersGlobal.vi" "Tracking Min Worm Area (Camera Pixels^2)"(w370) -> ()
      n227 = global write "ParametersGlobal.vi" "Tracking Smoothing Window (Camera Frames)"(w358) -> ()
      n228 = global write "ParametersGlobal.vi" "ParpoolTempIMAQArray"(w355) -> ()
      n229 = global write "ParametersGlobal.vi" "Tracking Mature Time (Camera Frames)"(w356) -> ()
      n230 = global write "ParametersGlobal.vi" "Tracking Max Backwards Time (Camera Frames)"(w346) -> ()
      n231 = call-dynamic "MakeExample.vi"("error in (no error)"=w344, "StimulusObject Parameters"="StimulusObject Parameters", "StimulusObject in"="StimulusObjectClassInput") -> ("error out"=w340:errorcluster, "StimulusObject out"=w349:refnum<class "StimulusObject.lvclass">)  [unwired: 7 in]
      n232 = global write "ParametersGlobal.vi" "Stimulus Example Object"(w349) -> ()
    }
  }
  n233 = Merge Errors(w10, w8) -> (→"error out":errorcluster)
